vi "startAgent.vi"(7 "daemon-config":T1={"resource-type"="battery", "agent-id"=12, "GA-ip"="192.168.1.1", "GA-port"=52020, "RA-ip"="127.0.0.1", "RA-port"=52001, "listenport-RA-side"=52011, "listenport-GA-side"=52021, "local-ip"="192.168.1.12", "long-term"=FALSE}) -> (0 "error out":errorcluster, 5 "connection ID":refnum<k16>)   [LabVIEW 2021]
uses:
  General purpose/daemon-config.ctl
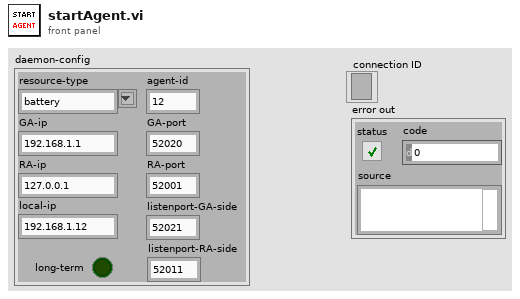
[diagram p1: front panel]
types:
  T1 = typedef "daemon-config.ctl" = cluster{"resource-type":string, "agent-id":u16, "GA-ip":string, "GA-port":u16, "RA-ip":string, "RA-port":u16, "listenport-RA-side":u16, "listenport-GA-side":u16, "local-ip":string, "long-term":bool}
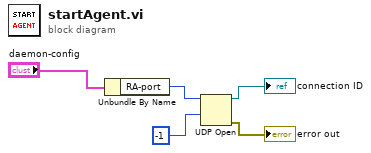
[diagram p0: block diagram]
diagram:
  n1 = Unbundle By Name("daemon-config") -> ("RA-port"=w3:u16)
  n2 = UDP Open(9:-1 ("timeout ms (25000)"), 11:w3) -> (port=→"connection ID":refnum<k16>, 0:→"error out":errorcluster)  [unwired: 3 in, 1 out]
